vi "defuerro.vi"(1 "active consequence":u8[](array[numeric])=[0], 2 "fullfilment consequence":dbl[](array[numeric]) format="%.2f", 3 "consequence":T1(array[cluster])=[{"ling.var."="out", "x-min"=-1.0, "x-max"=1.0, "setarray"=[{"linguistic term"="NEo", "color"=16711680, "points"=[-1.0, -1.0, -1.0, 0.0]}, {"linguistic term"="ZEo", "color"=255, "points"=[-1.0, 0.0, 0.0, 1.0]}, {"linguistic term"="POo", "color"=26214, "points"=[0.0, 1.0, 1.0, 1.0]}]}] {"x-min" format="%.2f"; "x-max" format="%.2f"; "setarray"."points" min=-1.0 max=1.0 step=0.10000000149011612 format="%.2f"}) -> (0 "error out":errorcluster={"status"=TRUE, "code"=15, "source"="too many/too\nless fullfilmentvalues"})   [LabVIEW 2017, in "NI_fuzzy logic.lvlib"]
uses:
  <vilib>/addons/control/fuzzy/NI_fuzzy logic.lvlib
panel:
  in  "error":errorcluster={"status"=TRUE, "code"=0, "source"=""}
  in  "no error":errorcluster
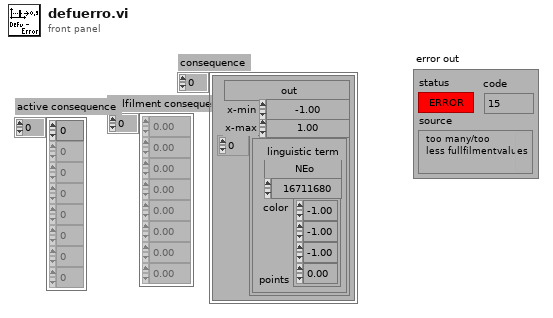
[diagram p1: front panel]
types:
  T1 = cluster{"ling.var.":string, "x-min":dbl, "x-max":dbl, "setarray":cluster{"linguistic term":string, "color":u32, "points":dbl[]}[]}[]
  T2 = cluster{"ling.var.":string, "x-min":dbl, "x-max":dbl, "setarray":cluster{"linguistic term":string, "color":u32, "points":dbl[]}[]}
  T3 = cluster{"linguistic term":string, "color":u32, "points":dbl[]}[]
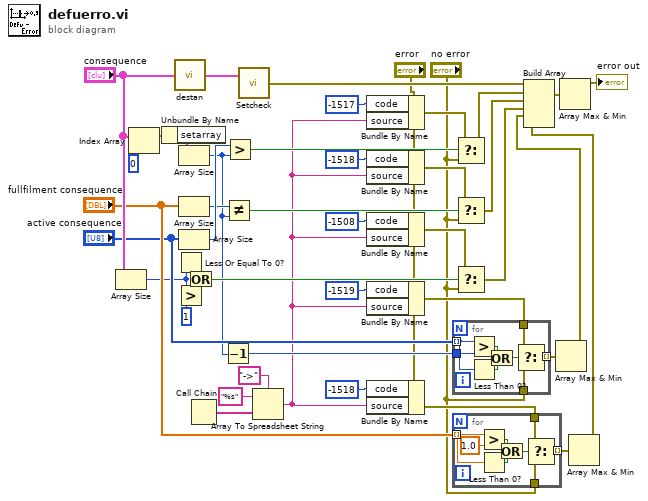
[diagram p0: block diagram]
diagram:
  n1 = Array Size(array="consequence") -> (size(s)=w38:i32)
  n2 = Index Array(array="consequence", index=0) -> (element=w35:T2)
  n3 = Unbundle By Name(w35) -> ("setarray"=w36:T3)
  n4 = call <vilib>:"destan.vi"("variablearray"="consequence") -> ("destandarized variable array"=w10:T1)
  n5 = Less Or Equal To 0?(x=w38) -> (x <= 0?=w39:bool)
  n6 = Greater?(x=w38, y=1) -> (0:w40:bool)
  n7 = Array Size(array=w36) -> (size(s)=w22:i32)
  n8 = Array Size(array="fullfilment consequence") -> (size(s)=w23:i32)
  n9 = Array Size(array="active consequence") -> (size(s)=w30:i32)
  n10 = Or(x=w39, y=w40) -> (x .or. y?=w41:bool)
  n11 = Call Chain() -> (call chain=w7:string[])
  n12 = Decrement(x=w22) -> (x-1=w31:i32)
  n13 = Not Equal?(x=w23, y=w22) -> (x != y?=w33:bool)
  n14 = Greater?(x=w30, y=w22) -> (0:w29:bool)
  n15 = call <vilib>:"Setcheck.vi"("variablearray"=w10) -> ("error out"=w27:errorcluster)  [unwired: 1 in]
  n16 = Array To Spreadsheet String(delimiter (Tab)="->", array=w7, 3:"%s" ("format string")) -> (spreadsheet string=w1:string)
  n17 = Bundle By Name(cluster="error", "code"=-1517, "source"=w1) -> (w25:errorcluster)
  n18 = Bundle By Name(cluster="error", "code"=-1518, "source"=w1) -> (w21:errorcluster)
  n19 = Bundle By Name(cluster="error", "code"=-1508, "source"=w1) -> (w18:errorcluster)
  n20 = Bundle By Name(cluster="error", "code"=-1519, "source"=w1) -> (w16:errorcluster)
  n21 = Bundle By Name(cluster="error", "code"=-1518, "source"=w1) -> (w14:errorcluster)
  n22 = for {
    tunnel: "active consequence" -> [w50] mode=indexing
    tunnel: w16 -> [w52]
    tunnel: w31 -> [w47]
    tunnel: [w51] -> w32 mode=indexing
    tunnel: "no error" -> [w45]
    n23 = Greater?(x=w50, y=w47) -> (0:w46:bool)
    n24 = Less Than 0?(x=w50) -> (x < 0?=w49:bool)
    n25 = Or(x=w46, y=w49) -> (x .or. y?=w48:bool)
    n26 = Select(t=w52, s=w48, f=w45) -> (s? t:f=w51:errorcluster)
  }
  n27 = for {
    tunnel: "fullfilment consequence" -> [w59] mode=indexing
    tunnel: [w60] -> w15 mode=indexing
    tunnel: w14 -> [w54]
    tunnel: "no error" -> [w53]
    n28 = Greater?(x=w59, y=1.0) -> (0:w56:bool)
    n29 = Less Than 0?(x=w59) -> (x < 0?=w55:bool)
    n30 = Or(x=w56, y=w55) -> (x .or. y?=w58:bool)
    n31 = Select(t=w54, s=w58, f=w53) -> (s? t:f=w60:errorcluster)
  }
  n32 = Select(t=w25, s=w29, f="no error") -> (s? t:f=w24:errorcluster)
  n33 = Select(t=w21, s=w33, f="no error") -> (s? t:f=w20:errorcluster)
  n34 = Select(t=w18, s=w41, f="no error") -> (s? t:f=w17:errorcluster)
  n35 = Array Max & Min(array=w32) -> (max value=w12:errorcluster)  [unwired: 3 out]
  n36 = Array Max & Min(array=w15) -> (max value=w11:errorcluster)  [unwired: 3 out]
  n37 = Build Array(w27, w24, w20, w17, w12, w11) -> (w28:errorcluster[])
  n38 = Array Max & Min(array=w28) -> (max value=→"error out":errorcluster)  [unwired: 3 out]
